vi "20190114_Filter_00_ATA_FPGA.vi"(4 "Probe 10":T2, 5 "EnableFIFO":bool, 6 "Scale":T1, 7 "output valid in":bool, 8 "Index":u32, 9 "Enable":T3, 10 "UnshiftedData":fxp<+/-,18,1>, 11 "ShiftedData":fxp<+/-,18,1>) -> (0 "Index out":u32, 1 "Probe 9":T2, 2 "fixed-point type":fxp<+/-,24,1>, 3 "output valid out":bool)   [LabVIEW 2018]
uses:
  FPGA_Controls/FPGA_Probe_Clust.ctl
  FPGA_Controls/FPGA_Enable_Clust.ctl
  FPGA_Controls/FPGA_Scale_Clust.ctl
  FPGA_Controls/FilterStageEnum.ctl
  <vilib>/rvi/FXPMathLib/FxpMul/XNode/nifxpmath_Multiplier.xnode
  <vilib>/rvi/FXPMathLib/sim/FxpSim.dll
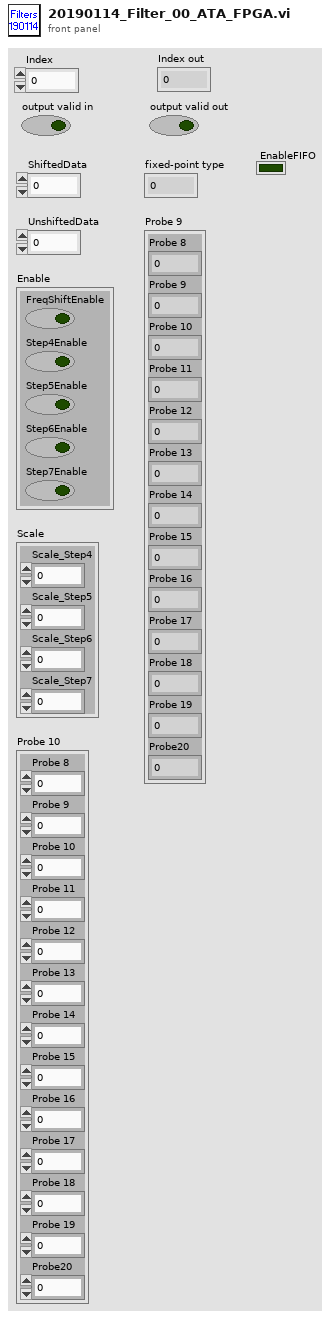
[diagram p1: front panel]
types:
  T1 = typedef "FPGA_Scale_Clust.ctl" = cluster{"Scale_Step4":fxp<+/-,23,23>, "Scale_Step5":fxp<+/-,23,23>, "Scale_Step6":fxp<+/-,23,23>, "Scale_Step7":fxp<+/-,23,23>}
  T2 = typedef "FPGA_Probe_Clust.ctl" = cluster{"Probe 8":fxp<+/-,18,1>, "Probe 9":fxp<+/-,24,1>, "Probe 10":fxp<+/-,24,1>, "Probe 11":fxp<+/-,24,1>, "Probe 12":fxp<+/-,47,24>, "Probe 13":fxp<+/-,24,1>, "Probe 14":fxp<+/-,25,2>, "Probe 15":fxp<+/-,48,25>, "Probe 16":fxp<+/-,24,1>, "Probe 17":fxp<+/-,25,2>, "Probe 18":fxp<+/-,48,25>, "Probe 19":fxp<+/-,24,1>, "Probe20":fxp<+/-,24,1>}
  T3 = typedef "FPGA_Enable_Clust.ctl" = cluster{"FreqShiftEnable":bool, "Step4Enable":bool, "Step5Enable":bool, "Step6Enable":bool, "Step7Enable":bool}
  T4 = typedef "FilterStageEnum.ctl" = enum16{"Digitiz0", "Digitiz1", "ScaleMeas", "Scale1", "Scale4", "Scale5", "Scale6", "Scale7"}
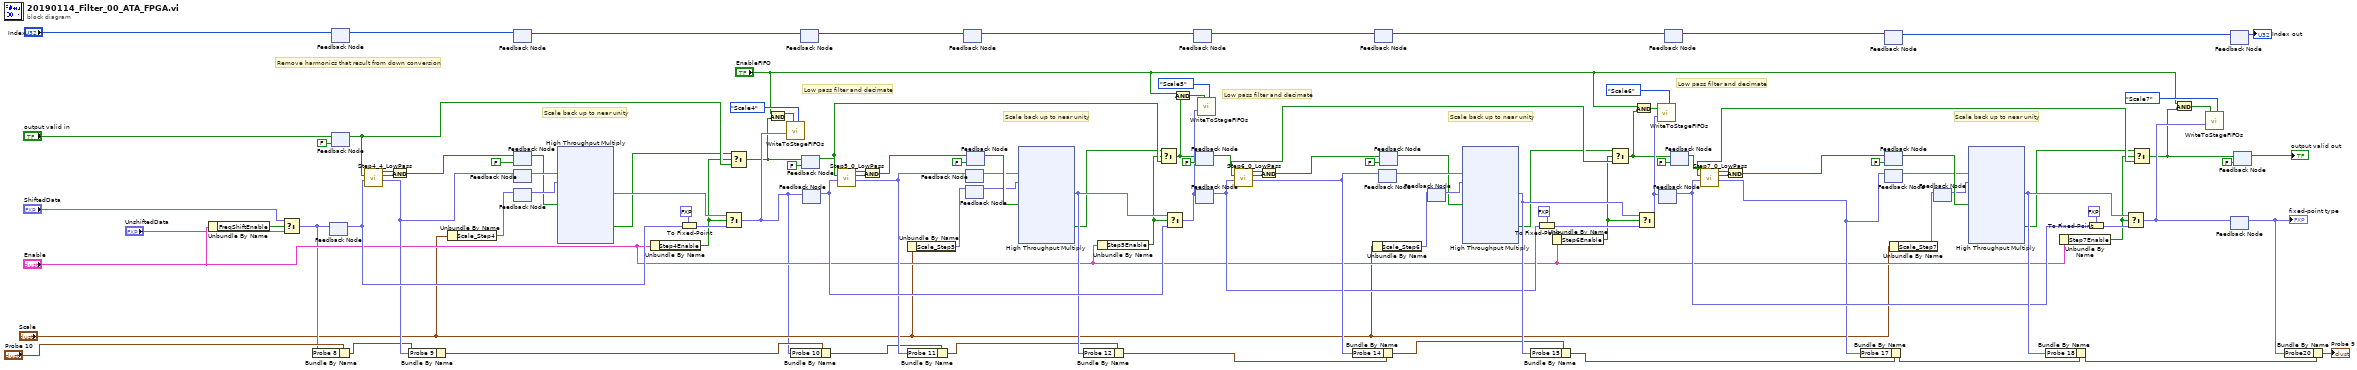
[diagram p0: block diagram]
diagram:
  # "Scale back up to near unity"
  # "Low pass filter and decimate"
  # "Scale back up to near unity"
  # "Low pass filter and decimate"
  # "Scale back up to near unity"
  # "Scale back up to near unity"
  # "Low pass filter and decimate"
  # "Remove harmonics that result from down conversion"
  n1 = Unbundle By Name("Enable") -> ("FreqShiftEnable"=w39:bool)
  n2 = Select(t="ShiftedData", s=w39, f="UnshiftedData") -> (s? t:f=w35:fxp<+/-,18,1>)
  n3 = Bundle By Name(cluster="Probe 10", "Probe 8"=w35) -> (w36:T2)
  n4 = feedback #1() -> (w95:fxp<+/-,18,1>)  [unwired: 1 in]
  n5 = feedback-in #1(w35) -> ()
  n6 = feedback #2() -> (w9:u32)  [unwired: 1 in]
  n7 = feedback-in #2("Index") -> ()
  n8 = feedback #3(FALSE ("output valid")) -> (w94:bool)
  n9 = feedback-in #3("output valid in") -> ()
  n10 = call "Step4_4_LowPass.vi"("s_axis_data_tdata"=w95, "s_axis_data_tvalid"=w94) -> ("m_axis_data_tdata"=w92:fxp<+/-,24,1>, "m_axis_data_tvalid"=w41:bool, "s_axis_data_tready"=w40:bool)  [unwired: 7 in]
  n11 = And(x=w40, y=w41) -> (x .and. y?=w93:bool)
  n12 = Bundle By Name(cluster=w36, "Probe 9"=w92) -> (w75:T2)
  n13 = Unbundle By Name("Scale") -> ("Scale_Step4"=w71:fxp<+/-,23,23>)
  n14 = feedback #4() -> (w8:u32)  [unwired: 1 in]
  n15 = feedback-in #4(w9) -> ()
  n16 = feedback #5(FALSE) -> (w42:bool)
  n17 = feedback-in #5(w93) -> ()
  n18 = feedback #6() -> (w44:fxp<+/-,24,1>)  [unwired: 1 in]
  n19 = feedback-in #6(w92) -> ()
  n20 = feedback #7() -> (w43:fxp<+/-,23,23>)  [unwired: 1 in]
  n21 = feedback-in #7(w71) -> ()
  n22 = xnode ("High Throughput Multiply")("x"=w44, "y"=w43, "input valid"=w42) -> ("x*y"=w91:fxp<+/-,24,1>, "output valid"=w90:bool)  [unwired: 1 in, 1 out]
  n23 = Unbundle By Name("Enable") -> ("Step4Enable"=w67:bool)
  n24 = To Fixed-Point(fixed-point type=fxp<+/-,24,1> 0.0, number=w95) -> (fixed-point=w89:fxp<+/-,24,1>)
  n25 = Select(t=w91, s=w67, f=w89) -> (s? t:f=w26:fxp<+/-,24,1>)
  n26 = Select(t=w90, s=w67, f=w94) -> (s? t:f=w18:bool)
  n27 = And(x="EnableFIFO", y=w18) -> (x .and. y?=w19:bool)
  n28 = call "WriteToStageFIFOs.vi"("Stage"=FilterStageEnum."Scale4", "Enable"=w19, "Scale4-7"=w26) -> ()  [unwired: 9 in]
  n29 = Bundle By Name(cluster=w75, "Probe 10"=w26) -> (w76:T2)
  n30 = feedback #8() -> (w7:u32)  [unwired: 1 in]
  n31 = feedback-in #8(w8) -> ()
  n32 = feedback #9(FALSE ("output valid")) -> (w100:bool)
  n33 = feedback-in #9(w18) -> ()
  n34 = feedback #10() -> (w99:fxp<+/-,24,1>)  [unwired: 1 in]
  n35 = feedback-in #10(w26) -> ()
  n36 = call "Step5_0_LowPass.vi"("s_axis_data_tdata"=w99, "s_axis_data_tvalid"=w100) -> ("m_axis_data_tdata"=w98:fxp<+/-,24,1>, "m_axis_data_tvalid"=w48:bool, "s_axis_data_tready"=w49:bool)  [unwired: 7 in]
  n37 = And(x=w49, y=w48) -> (x .and. y?=w101:bool)
  n38 = Unbundle By Name("Scale") -> ("Scale_Step5"=w72:fxp<+/-,23,23>)
  n39 = Bundle By Name(cluster=w76, "Probe 11"=w98) -> (w77:T2)
  n40 = feedback #11() -> (w6:u32)  [unwired: 1 in]
  n41 = feedback-in #11(w7) -> ()
  n42 = feedback #12() -> (w45:fxp<+/-,24,1>)  [unwired: 1 in]
  n43 = feedback-in #12(w98) -> ()
  n44 = feedback #13() -> (w46:fxp<+/-,23,23>)  [unwired: 1 in]
  n45 = feedback-in #13(w72) -> ()
  n46 = feedback #14(FALSE ("output valid")) -> (w47:bool)
  n47 = feedback-in #14(w101) -> ()
  n48 = xnode ("High Throughput Multiply")("x"=w45, "y"=w46, "input valid"=w47) -> ("x*y"=w97:fxp<+/-,24,1>, "output valid"=w96:bool)  [unwired: 1 in, 1 out]
  n49 = Bundle By Name(cluster=w77, "Probe 12"=w97) -> (w78:T2)
  n50 = Unbundle By Name("Enable") -> ("Step5Enable"=w68:bool)
  n51 = Select(t=w96, s=w68, f=w100) -> (s? t:f=w16:bool)
  n52 = Select(t=w97, s=w68, f=w99) -> (s? t:f=w24:fxp<+/-,24,1>)
  n53 = And(x="EnableFIFO", y=w16) -> (x .and. y?=w17:bool)
  n54 = feedback #15() -> (w5:u32)  [unwired: 1 in]
  n55 = feedback-in #15(w6) -> ()
  n56 = feedback #16(FALSE ("output valid")) -> (w104:bool)
  n57 = feedback-in #16(w16) -> ()
  n58 = feedback #17() -> (w105:fxp<+/-,24,1>)  [unwired: 1 in]
  n59 = feedback-in #17(w24) -> ()
  n60 = call "WriteToStageFIFOs.vi"("Stage"=FilterStageEnum."Scale5", "Enable"=w17, "Scale4-7"=w24) -> ()  [unwired: 9 in]
  n61 = call "Step6_0_LowPass.vi"("s_axis_data_tdata"=w105, "s_axis_data_tvalid"=w104) -> ("m_axis_data_tdata"=w108:fxp<+/-,24,2>, "m_axis_data_tvalid"=w51:bool, "s_axis_data_tready"=w50:bool)  [unwired: 7 in]
  n62 = And(x=w50, y=w51) -> (x .and. y?=w107:bool)
  n63 = Bundle By Name(cluster=w78, "Probe 14"=w108) -> (w79:T2)
  n64 = Unbundle By Name("Scale") -> ("Scale_Step6"=w73:fxp<+/-,23,23>)
  n65 = feedback #18() -> (w4:u32)  [unwired: 1 in]
  n66 = feedback-in #18(w5) -> ()
  n67 = feedback #19() -> (w53:fxp<+/-,24,2>)  [unwired: 1 in]
  n68 = feedback-in #19(w108) -> ()
  n69 = feedback #20(FALSE ("output valid")) -> (w52:bool)
  n70 = feedback-in #20(w107) -> ()
  n71 = feedback #21() -> (w54:fxp<+/-,23,23>)  [unwired: 1 in]
  n72 = feedback-in #21(w73) -> ()
  n73 = xnode ("High Throughput Multiply")("x"=w53, "y"=w54, "input valid"=w52) -> ("x*y"=w106:fxp<+/-,24,1>, "output valid"=w103:bool)  [unwired: 1 in, 1 out]
  n74 = Bundle By Name(cluster=w79, "Probe 15"=w106) -> (w80:T2)
  n75 = To Fixed-Point(fixed-point type=fxp<+/-,24,1> 0.0, number=w105) -> (fixed-point=w84:fxp<+/-,24,1>)
  n76 = Unbundle By Name("Enable") -> ("Step6Enable"=w69:bool)
  n77 = Select(t=w103, s=w69, f=w104) -> (s? t:f=w14:bool)
  n78 = And(x="EnableFIFO", y=w14) -> (x .and. y?=w15:bool)
  n79 = Select(t=w106, s=w69, f=w84) -> (s? t:f=w22:fxp<+/-,24,1>)
  n80 = call "WriteToStageFIFOs.vi"("Stage"=FilterStageEnum."Scale6", "Enable"=w15, "Scale4-7"=w22) -> ()  [unwired: 9 in]
  n81 = feedback #22() -> (w113:fxp<+/-,24,1>)  [unwired: 1 in]
  n82 = feedback-in #22(w22) -> ()
  n83 = feedback #23() -> (w3:u32)  [unwired: 1 in]
  n84 = feedback-in #23(w4) -> ()
  n85 = feedback #24(FALSE ("output valid")) -> (w112:bool)
  n86 = feedback-in #24(w14) -> ()
  n87 = call "Step7_0_LowPass.vi"("s_axis_data_tdata"=w113, "s_axis_data_tvalid"=w112) -> ("m_axis_data_tdata"=w109:fxp<+/-,24,2>, "m_axis_data_tvalid"=w58:bool, "s_axis_data_tready"=w59:bool)  [unwired: 7 in]
  n88 = And(x=w59, y=w58) -> (x .and. y?=w110:bool)
  n89 = Bundle By Name(cluster=w80, "Probe 17"=w109) -> (w81:T2)
  n90 = feedback #25() -> (w56:fxp<+/-,24,2>)  [unwired: 1 in]
  n91 = feedback-in #25(w109) -> ()
  n92 = feedback #26() -> (w2:u32)  [unwired: 1 in]
  n93 = feedback-in #26(w3) -> ()
  n94 = feedback #27(FALSE ("output valid")) -> (w57:bool)
  n95 = feedback-in #27(w110) -> ()
  n96 = Unbundle By Name("Scale") -> ("Scale_Step7"=w74:fxp<+/-,23,23>)
  n97 = feedback #28() -> (w55:fxp<+/-,23,23>)  [unwired: 1 in]
  n98 = feedback-in #28(w74) -> ()
  n99 = xnode ("High Throughput Multiply")("x"=w56, "y"=w55, "input valid"=w57) -> ("x*y"=w114:fxp<+/-,24,1>, "output valid"=w111:bool)  [unwired: 1 in, 1 out]
  n100 = Bundle By Name(cluster=w81, "Probe 18"=w114) -> (w82:T2)
  n101 = Unbundle By Name("Enable") -> ("Step7Enable"=w70:bool)
  n102 = To Fixed-Point(fixed-point type=fxp<+/-,24,1> 0.0, number=w113) -> (fixed-point=w87:fxp<+/-,24,1>)
  n103 = Select(t=w114, s=w70, f=w87) -> (s? t:f=w20:fxp<+/-,24,1>)
  n104 = Select(t=w111, s=w70, f=w112) -> (s? t:f=w11:bool)
  n105 = And(x="EnableFIFO", y=w11) -> (x .and. y?=w12:bool)
  n106 = call "WriteToStageFIFOs.vi"("Stage"=FilterStageEnum."Scale7", "Enable"=w12, "Scale4-7"=w20) -> ()  [unwired: 9 in]
  n107 = feedback #29() -> (→"Index out":u32)  [unwired: 1 in]
  n108 = feedback-in #29(w2) -> ()
  n109 = feedback #30() -> (w29:fxp<+/-,24,1>)  [unwired: 1 in]
  "fixed-point type" <- w29
  n110 = feedback-in #30(w20) -> ()
  n111 = feedback #31(FALSE ("output valid")) -> (→"output valid out":bool)
  n112 = feedback-in #31(w11) -> ()
  n113 = Bundle By Name(cluster=w82, "Probe20"=w29) -> (→"Probe 9":T2)
